vi "GetMethodExecutionInfoByName.vi"(0 "Executer in":refnum<class "Executer.lvclass">, 2 "Class in":string, 3 "Method":string, 5 "error in (no error)":errorcluster) -> (14 "Executer out":refnum<class "Executer.lvclass">, 16 "Class":refnum<class>, 17 "Method":T1, 19 "error out":errorcluster)   [LabVIEW 2018, in "Executer.lvclass"]
uses:
  Executer.lvclass
  typedefs/MethodExecutionInfo.ctl
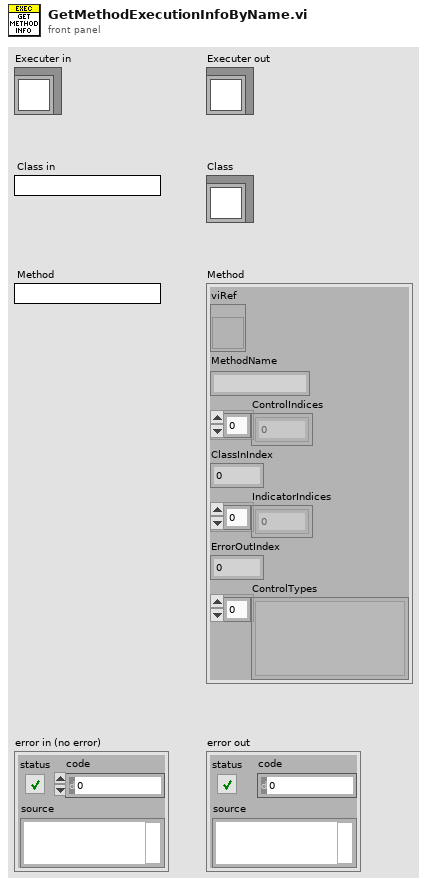
[diagram p1: front panel]
types:
  T1 = typedef "Executer.lvclass/MethodExecutionInfo.ctl" = cluster{"viRef":refnum<vi>, "MethodName":string, "ControlIndices":i32[], "ClassInIndex":i32, "IndicatorIndices":i32[], "ErrorOutIndex":i32, "ControlTypes":variant[]}
  T2 = typedef "Executer.lvclass/ObjectAttributes.ctl" = cluster{"Executions":T3[]}
  T3 = typedef "Executer.lvclass/ClassExecutionInfo.ctl" = cluster{"Class":refnum<class>, "ClassName":string, "VIExecutionInfo":T1[]}
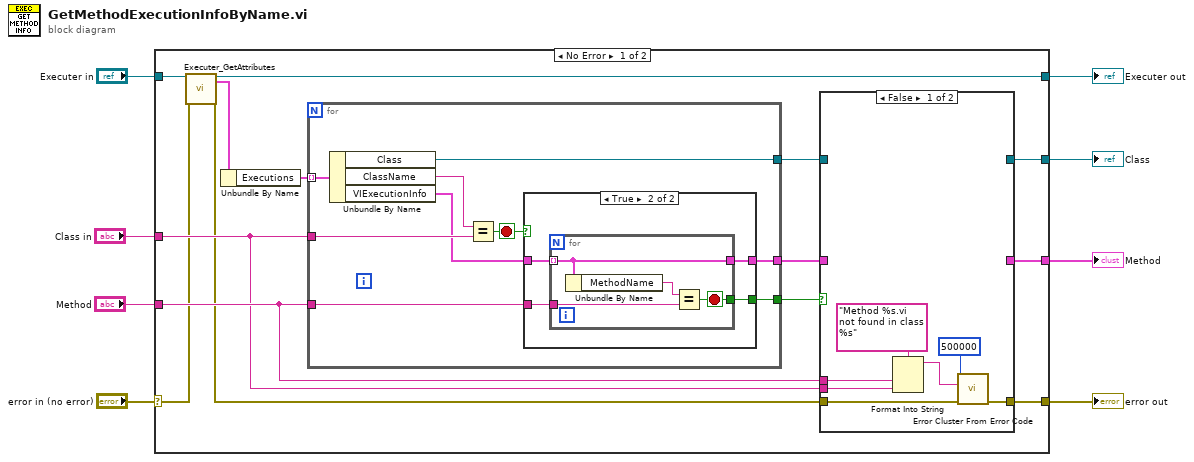
[diagram p0: block diagram]
diagram:
  n1 = case shown="No Error" "error in (no error)" {
    selector: "error in (no error)" -> [w9 w50]
    tunnel: [w21 w51] -> w8
    tunnel: "Executer in" -> [w20 w51]
    tunnel: "Method" -> [w17 _]
    tunnel: "Class in" -> [w16 _]
    tunnel: [w14 w50] -> w4
    tunnel: [w11 _] -> w3
    tunnel: [w10 _] -> w2
    frame No Error {
      n2 = call "Executer_GetAttributes.vi"("reference in"=w20, "error in (no error)"=w9) -> ("reference out"=w21:refnum<class "Executer.lvclass">, "Data"=w19:T2, "error out"=w15:errorcluster)  [unwired: 14 in, 1 out]
      n3 = Unbundle By Name(w19) -> ("Executions"=w22:T3[])
      n4 = for {
        tunnel: w22 -> [w41] mode=indexing
        tunnel: w16 -> [w38]
        tunnel: [w39] -> w12
        tunnel: w17 -> [w37]
        tunnel: [w36] -> w18
        tunnel: [w33] -> w13
        stop <- w40 stop-if-true
        n5 = Unbundle By Name(w41) -> ("Class"=w33:refnum<class>, "ClassName"=w35:string, "VIExecutionInfo"=w34:T1[])
        n6 = Equal?(x=w35, y=w38) -> (x = y?=w40:bool)
        n7 = case shown="True" w40 {
          tunnel: w34 -> [_ w45]
          tunnel: [_ w44] -> w39
          tunnel: w37 -> [_ w43]
          tunnel: [_ w42] -> w36
          frame False {
          }
          frame True {
            n8 = for {
              tunnel: w45 -> [w49] mode=indexing
              tunnel: [w49] -> w44
              tunnel: w43 -> [w47]
              tunnel: [w46] -> w42
              stop <- w46 stop-if-true
              n9 = Unbundle By Name(w49) -> ("MethodName"=w48:string)
              n10 = Equal?(x=w48, y=w47) -> (x = y?=w46:bool)
            }
          }
        }
      }
      n11 = case shown="False" w18 {
        tunnel: w17 -> [w26 _]
        tunnel: w16 -> [w25 _]
        tunnel: w15 -> [w24 w30]
        tunnel: [w23 w30] -> w14
        tunnel: [_ w32] -> w10
        tunnel: w13 -> [_ w32]
        tunnel: [_ w31] -> w11
        tunnel: w12 -> [_ w31]
        frame False {
          n12 = Format Into String(format string="Method %s.vi not found in class %s", w26, w25) -> (resulting string=w28:string)  [unwired: 2 in, 1 out]
          n13 = call <vilib>:"Error Cluster From Error Code.vi"("error in (no error)"=w24, "error message (\"\")"=w28, "error code (0)"=500000) -> ("error out"=w23:errorcluster)  [unwired: 6 in]
        }
        frame True {
        }
      }
    }
    frame Error {
    }
  }
  "Class" <- w2
  "error out" <- w4
  "Method" <- w3
  "Executer out" <- w8
